vi "MessageName.vi"() -> (2 "MessageName":string)   [LabVIEW 2020, in "DoubleData.lvlib"]
uses:
  DoubleData.lvlib
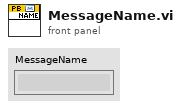
[diagram p1: front panel]
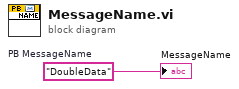
[diagram p0: block diagram]
diagram:
  w1 = "DoubleData"  # PB MessageName
  "MessageName" <- w1
